vi "p00 - For Loop and Timer.vi"() -> ()   [LabVIEW 2025]
uses:
  <vilib>/numeric/Random Number (Range) U64.vi
  <vilib>/numeric/sub_Random U32.vi
panel:
  in  "Start":bool
  out "Random Number":u64
  in  "Wait (ms)":u32=500
  in  "Iteration Amount":i32=10
  out "Iteration Count":i32
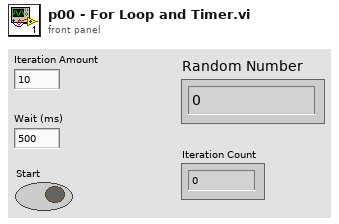
[diagram p1: front panel]
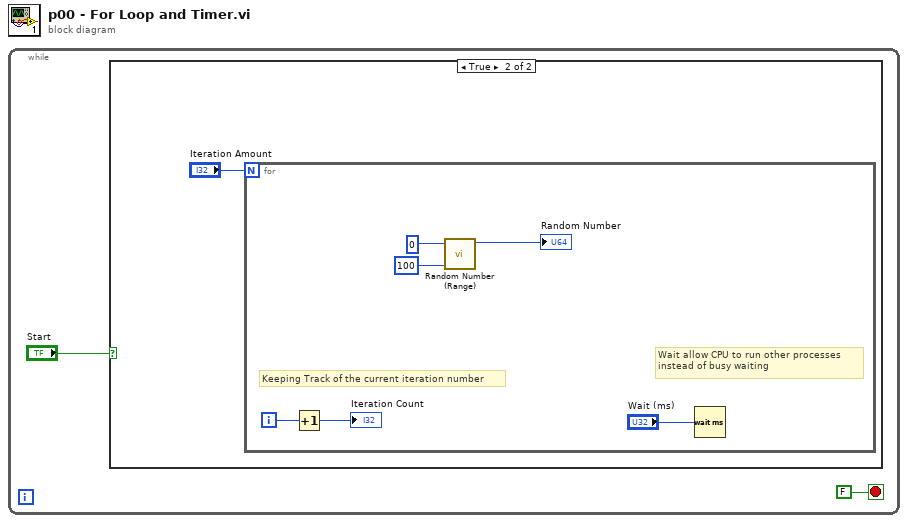
[diagram p0: block diagram]
diagram:
  n1 = while {
    stop <- FALSE stop-if-true
    n2 = case shown="True" "Start" {
      frame False {
      }
      frame True {
        n3 = for {
          N: "Iteration Amount" -> [_]
          i -> [w5]
          # "Keeping Track of the current iteration number"
          # "Wait allow CPU to run other processes \ninstead of busy waiting"
          n4 = Increment(x=w5) -> (x+1=→"Iteration Count":i32)
          n5 = call-poly <vilib>:"Random Number (Range).vi"("lower bound (0)"=u64 0, "upper bound (100)"=u64 100) -> ("number"=→"Random Number":u64)  [unwired: 9 in]
          n6 = Wait (ms)(milliseconds to wait="Wait (ms)") -> ()  [unwired: 1 out]
        }
      }
    }
  }
